vi "Comments.vi"   [LabVIEW 2019]
panel:
  # "Comment1"
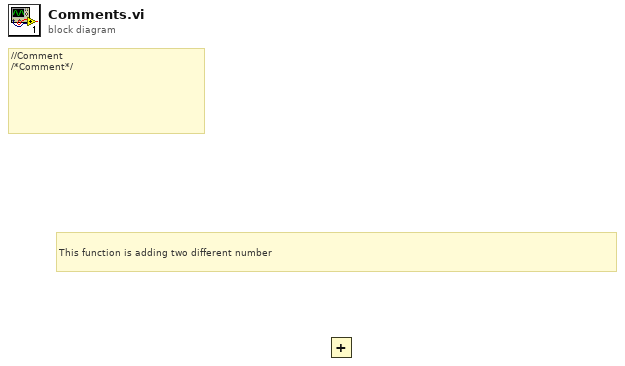
[diagram p0: block diagram]
diagram:
  # "This function is adding two different number"
  # "//Comment\n/*Comment*/"
  n1 = Add() -> ()  [unwired: 2 in, 1 out]
